vi "function.vi"(9 "Y":dbl, 11 "X":dbl) -> (2 "Z(x, y)":dbl)   [LabVIEW 2026]
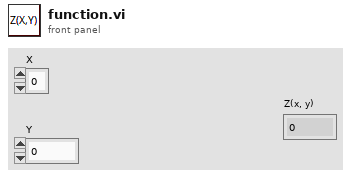
[diagram p1: front panel]
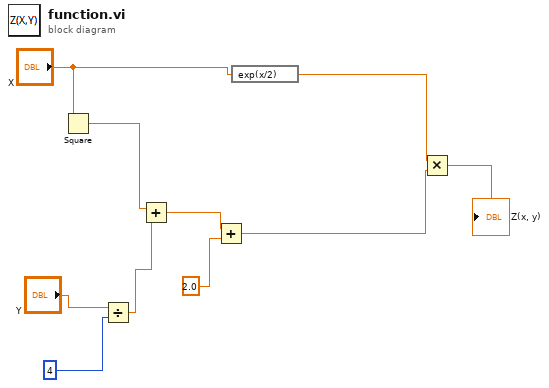
[diagram p0: block diagram]
diagram:
  n1 = Square(x="X") -> (x^2=w4:dbl)
  n2 = Divide(x="Y", y=4) -> (x/y=w6:dbl)
  n3 = Add(x=w4, y=w6) -> (x+y=w3:dbl)
  n4 = Add(x=w3, y=2.0) -> (x+y=w5:dbl)
  n5 = expression code="exp(x/2)"("X") -> (w9:dbl)
  n6 = Multiply(x=w9, y=w5) -> (x*y=→"Z(x, y)":dbl)
